vi "Inst_CNT90.vi"(8 "error in":errorcluster, 10 "All Message Queues in":T1, 11 "Prueba31 in":refnum<class "Prueba31.lvclass">) -> (0 "error out":errorcluster)   [LabVIEW 2019, in "Prueba31.lvclass"]
uses:
  Prueba31.lvclass
  QMH/Message Queue/All Message Queues.ctl
  QMH/Message Queue/Message Cluster.ctl
  Prueba31.lvclass/Prueba31.ctl
  <vilib>/Utility/error.llb/Error Cluster From Error Code.vi
  QMH/Message Queue/Enqueue Message (Single).vi
  <vilib>/ErrorRing/Error Ring.xnode
  QMH/Message Queue/Message Queue.lvlib
  Instrumento/CNT90/CNT90.lvclass
panel:
  out "All States":string[](array[string])
  out "Actual State":string
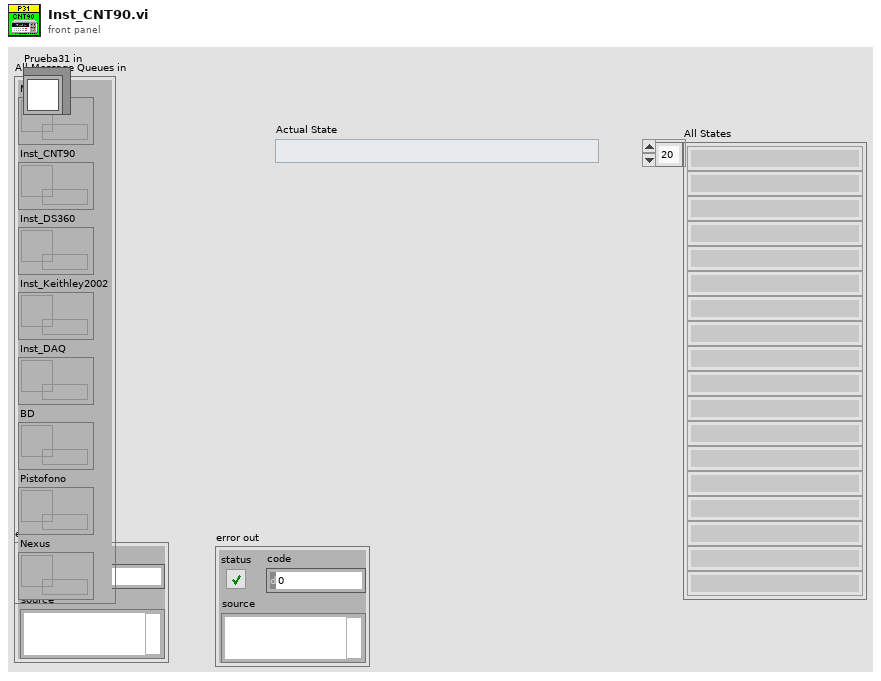
[diagram p1: front panel]
types:
  T1 = typedef "Message Queue.lvlib/All Message Queues.ctl" = cluster{"MHL":refnum<queue>, "Inst_CNT90":refnum<queue>, "Inst_DS360":refnum<queue>, "Inst_Keithley2002":refnum<queue>, "Inst_DAQ":refnum<queue>, "BD":refnum<queue>, "Pistofono":refnum<queue>, "Nexus":refnum<queue>}
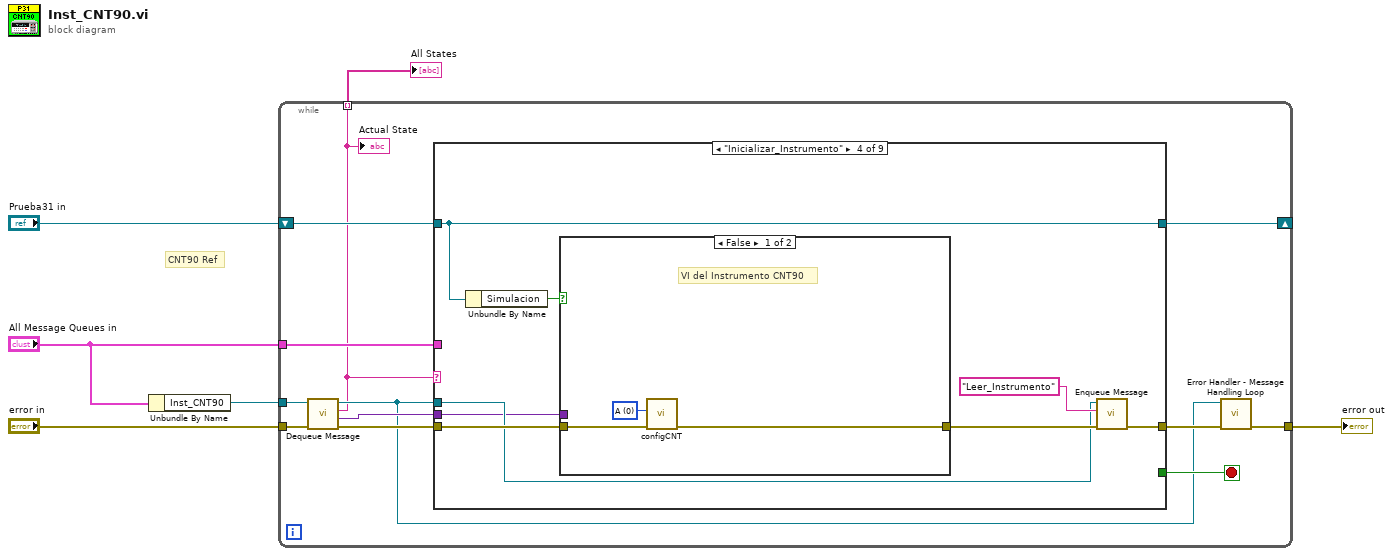
[diagram p0: block diagram]
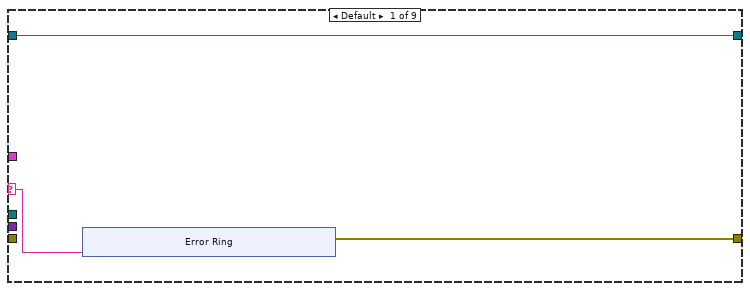
[diagram p2: hidden frame]
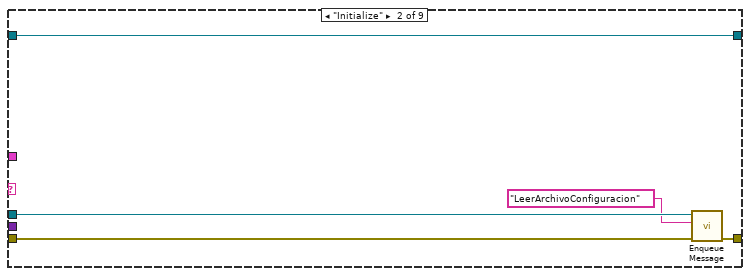
[diagram p3: hidden frame]
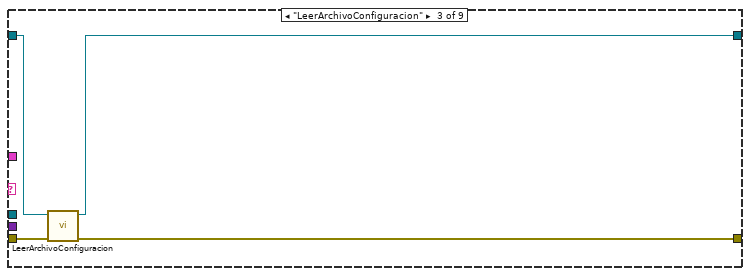
[diagram p4: hidden frame]
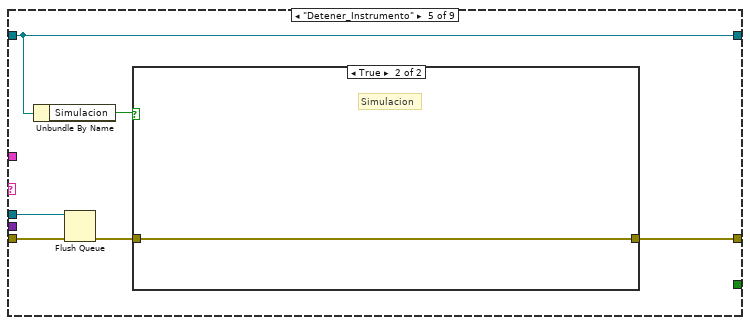
[diagram p6: hidden frame]
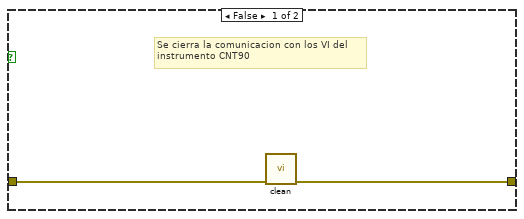
[diagram p7: hidden frame]
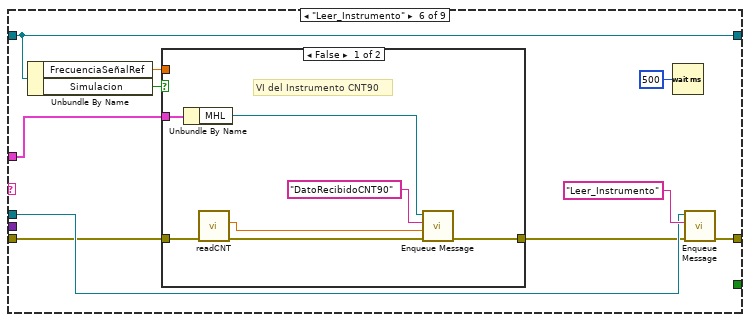
[diagram p8: hidden frame]
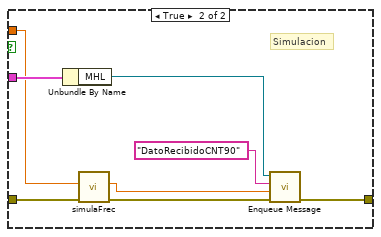
[diagram p9: hidden frame]
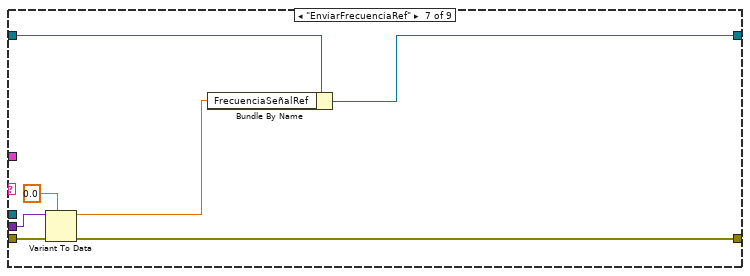
[diagram p10: hidden frame]
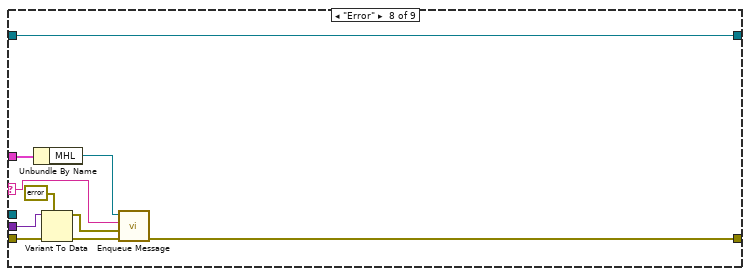
[diagram p11: hidden frame]
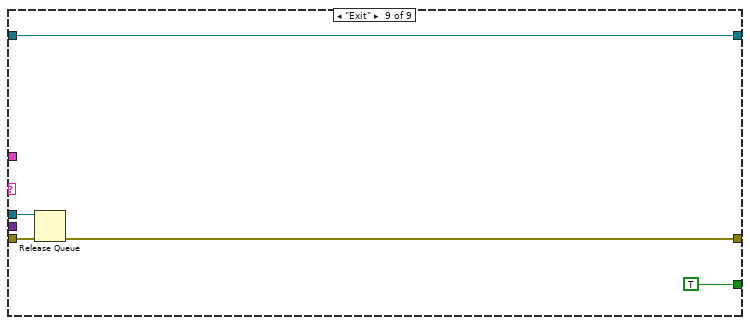
[diagram p12: hidden frame]
diagram:
  # "CNT90 Ref"
  n1 = Unbundle By Name("All Message Queues in") -> ("Inst_CNT90"=w4:refnum<queue>)
  n2 = while {
    tunnel: "error in" -> [w18]
    tunnel: w4 -> [w17]
    tunnel: "All Message Queues in" -> [w16]
    tunnel: [w9] -> w2
    shift-right: [w12] -> _
    shift-left: "Prueba31 in" -> [w15]
    tunnel: [w7] -> w1 mode=indexing
    stop <- w11 stop-if-true
    n3 = call "Dequeue Message.vi"("error in (no error)"=w18, "Message Queue"=w17) -> ("error out"=w13:errorcluster, "Message Data"=w14:variant, "Message"=w7:string, "dup Message Queue"=w8:refnum<queue>)  [unwired: 6 in]
    "Actual State" <- w7
    n4 = case shown="\"Inicializar_Instrumento\"" w7 {
      selector: w7 -> [w21 _ _ _ _ _ _ w95 _]
      tunnel: w16 -> [_ _ _ _ _ w60 _ w94 _]
      tunnel: w15 -> [w19 w33 w34 w45 w54 w62 w85 w92 w102]
      tunnel: w8 -> [_ w30 _ w39 w50 w66 _ _ w104]
      tunnel: w14 -> [_ _ _ w38 _ _ w88 w98 _]
      tunnel: w13 -> [_ w31 w35 w44 w51 w64 w89 w99 w105]
      tunnel: [w20 w32 w37 w41 w55 w67 w90 w91 w101] -> w10
      tunnel: [w19 w33 w36 w45 w54 w62 w86 w92 w102] -> w12
      tunnel: [_ _ _ _ _ _ _ _ TRUE] -> w11
      frame Default {
        n5 = xnode "Error Ring"("parameter 0"=w21) -> ("error out"=w20:errorcluster)
      }
      frame "Initialize" {
        n6 = call-poly "Enqueue Message.vi"("error in (no error)"=w31, "Message"="LeerArchivoConfiguracion", "Message Queue"=w30) -> ("error out"=w32:errorcluster)  [unwired: 7 in, 1 out]
      }
      frame "LeerArchivoConfiguracion" {
        n7 = call "LeerArchivoConfiguracion.vi"("error in"=w35, "Prueba31 in"=w34) -> ("error out"=w37:errorcluster, "Prueba31 out"=w36:refnum<class "Prueba31.lvclass">)  [unwired: 8 in]
      }
      frame "Inicializar_Instrumento" {
        n8 = Unbundle By Name(w45) -> ("Simulacion"=w43:bool)
        n9 = case shown="False" w43 {
          tunnel: [w48 w49] -> w40
          tunnel: w44 -> [w47 w49]
          tunnel: w38 -> [_ _]
          frame False {
            w46 = 0 items=["A", "B"] ("Channel  1")
            # "VI del Instrumento CNT90"
            n10 = call "configCNT.vi"("error in (no error)"=w47, "Channel  1"=w46) -> ("error out"=w48:errorcluster)  [unwired: 8 in, 1 out]
          }
          frame True {
            # "Simulacion"
          }
        }
        n11 = call-poly "Enqueue Message.vi"("error in (no error)"=w40, "Message"="Leer_Instrumento", "Message Queue"=w39) -> ("error out"=w41:errorcluster)  [unwired: 7 in, 1 out]
      }
      frame "Detener_Instrumento" {
        n12 = Unbundle By Name(w54) -> ("Simulacion"=w53:bool)
        n13 = Flush Queue(queue=w50, error in (no error)=w51) -> (error out=w52:errorcluster)  [unwired: 2 out]
        n14 = case shown="True" w53 {
          tunnel: [w57 w58] -> w55
          tunnel: w52 -> [w56 w58]
          frame False {
            # "Se cierra la comunicacion con los VI del\ninstrumento CNT90"
            n15 = call "clean.vi"("error in (no error)"=w56) -> ("error out"=w57:errorcluster)  [unwired: 9 in, 1 out]
          }
          frame True {
            # "Simulacion"
          }
        }
      }
      frame "Leer_Instrumento" {
        n16 = Unbundle By Name(w62) -> ("FrecuenciaSeñalRef"=w59:dbl, "Simulacion"=w61:bool)
        n17 = case shown="False" w61 {
          tunnel: [w72 w82] -> w63
          tunnel: w64 -> [w75 w79]
          tunnel: w60 -> [w71 w81]
          tunnel: w59 -> [_ w76]
          frame False {
            # "VI del Instrumento CNT90"
            n18 = Unbundle By Name(w71) -> ("MHL"=w70:refnum<queue>)
            n19 = call "readCNT.vi"("error in (no error)"=w75) -> ("error out"=w73:errorcluster, "medicion"=w69:dbl)  [unwired: 8 in, 1 out]
            n20 = call-poly "Enqueue Message.vi"("error in (no error)"=w73, "Message Data"=w69, "Message"="DatoRecibidoCNT90", "Message Queue"=w70) -> ("error out"=w72:errorcluster)  [unwired: 6 in, 1 out]
          }
          frame True {
            # "Simulacion"
            n21 = Unbundle By Name(w81) -> ("MHL"=w80:refnum<queue>)
            n22 = call "simulaFrec.vi"("error in (no error)"=w79, "frec in"=w76) -> ("error out"=w78:errorcluster, "frec out"=w77:dbl)  [unwired: 7 in, 1 out]
            n23 = call-poly "Enqueue Message.vi"("error in (no error)"=w78, "Message Data"=w77, "Message"="DatoRecibidoCNT90", "Message Queue"=w80) -> ("error out"=w82:errorcluster)  [unwired: 6 in, 1 out]
          }
        }
        n24 = Wait (ms)(milliseconds to wait=u32 500) -> ()  [unwired: 1 out]
        n25 = call-poly "Enqueue Message.vi"("error in (no error)"=w63, "Message"="Leer_Instrumento", "Message Queue"=w66) -> ("error out"=w67:errorcluster)  [unwired: 7 in, 1 out]
      }
      frame "EnviarFrecuenciaRef" {
        n26 = Variant To Data(error in=w89, type=0.0, Variant=w88) -> (data=w84:dbl, error out=w90:errorcluster)
        n27 = Bundle By Name(cluster=w85, "FrecuenciaSeñalRef"=w84) -> (w86:refnum<class "Prueba31.lvclass">)
      }
      frame "Error" {
        n28 = Unbundle By Name(w94) -> ("MHL"=w93:refnum<queue>)
        n29 = Variant To Data(error in=w99, type=errorcluster {"status"=FALSE, "code"=0, "source"=""} ("error constant"), Variant=w98) -> (data=w96:errorcluster, error out=w97:errorcluster)
        n30 = call-poly "Enqueue Message.vi"("error in (no error)"=w97, "Message Data"=w96, "Message"=w95, "Message Queue"=w93) -> ("error out"=w91:errorcluster)  [unwired: 6 in, 1 out]
      }
      frame "Exit" {
        n31 = Release Queue(queue=w104, error in (no error)=w105) -> (error out=w101:errorcluster)  [unwired: 1 in, 2 out]
      }
    }
    n32 = call "Error Handler - Message Handling Loop.vi"("error in (no error)"=w10, "Message Queue"=w8) -> ("dup error in"=w9:errorcluster)  [unwired: 8 in, 1 out]
  }
  "error out" <- w2
  "All States" <- w1
